vi "Configure Frequency Response Analysis Characteristics.vi"(5 "Enable Amplitude Ramp (F: Disable)":bool, 6 "Trace (4: Gain and Phase)":i32(ring)=4 items=["None", "All", "Gain", "Phase", "Gain and Phase"], 7 "Point Number (10: 10)":i32(ring)=10 items=["10"=10, "20"=20, "30"=30, "40"=40, "50"=50, "60"=60, "70"=70, "80"=80, "90"=90, "100"=100], 8 "error in (no error)":errorcluster, 9 "Single Frequency Value (1: 100 Hz)":i32(ring)=1 items=["20", "100", "1000", "10000", "100000", "1000000", "10000000", "2000000", "10"], 10 "Frequency Mode (0: Sweep)":i32(ring) items=["Sweep", "Single"], 11 "VISA resource name":refnum<visa-resource-name>) -> (0 "error out":errorcluster, 3 "VISA resource name out":refnum<visa-resource-name>)   [LabVIEW 2015, in "Agilent 2000 3000 X-Series.lvlib"]
doc: "Configure frequency response analysis feature.\n\n<b>Note:</b>\nThis VI is only applicable for 3000T, 4000, 6000 X-Series, 1000 X-Series after 1.10 firmware"
uses:
  Agilent 2000 3000 X-Series.lvlib
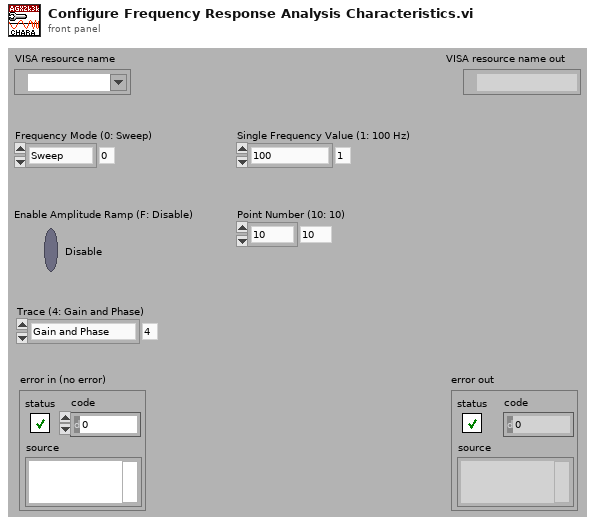
[diagram p1: front panel]
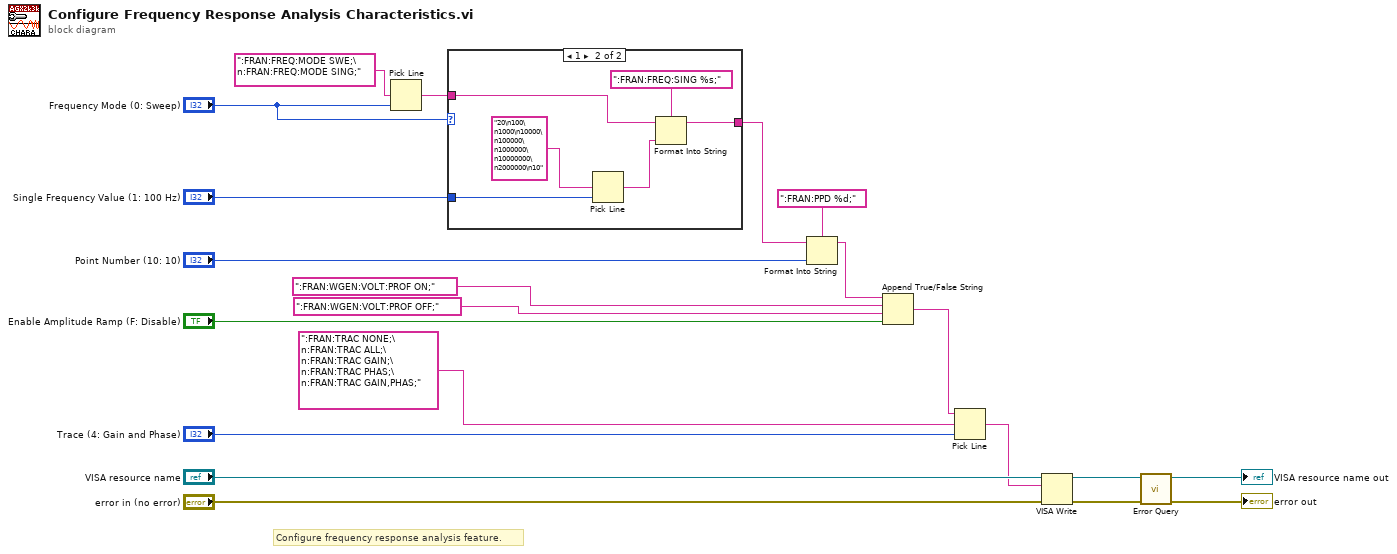
[diagram p0: block diagram]
diagram:
  # "Configure frequency response analysis feature."
  n1 = Pick Line(multi-line string=":FRAN:FREQ:MODE SWE;\n:FRAN:FREQ:MODE SING;", line index="Frequency Mode (0: Sweep)") -> (output string=w9:string)  [unwired: 1 in]
  n2 = case shown="1" "Frequency Mode (0: Sweep)" {
    tunnel: w9 -> [w22 w27]
    tunnel: [w22 w26] -> w8
    tunnel: "Single Frequency Value (1: 100 Hz)" -> [_ w23]
    frame 0, Default {
    }
    frame 1 {
      n3 = Pick Line(multi-line string="20\n100\n1000\n10000\n100000\n1000000\n10000000\n2000000\n10", line index=w23) -> (output string=w25:string)  [unwired: 1 in]
      n4 = Format Into String(format string=":FRAN:FREQ:SING %s;", initial string=w27, w25) -> (resulting string=w26:string)  [unwired: 1 in, 1 out]
    }
  }
  n5 = Format Into String(format string=":FRAN:PPD %d;", initial string=w8, "Point Number (10: 10)") -> (resulting string=w7:string)  [unwired: 1 in, 1 out]
  n6 = Append True/False String(1:"Enable Amplitude Ramp (F: Disable)", 2:":FRAN:WGEN:VOLT:PROF OFF;", 3:":FRAN:WGEN:VOLT:PROF ON;", 4:w7) -> (0:w4:string)
  n7 = Pick Line(string ("")=w4, multi-line string=":FRAN:TRAC NONE;\n:FRAN:TRAC ALL;\n:FRAN:TRAC GAIN;\n:FRAN:TRAC PHAS;\n:FRAN:TRAC GAIN,PHAS;", line index="Trace (4: Gain and Phase)") -> (output string=w3:string)
  n8 = VISA Write(VISA resource name="VISA resource name", write buffer=w3, error in (no error)="error in (no error)") -> (VISA resource name out=w14:refnum<visa-resource-name>, error out=w13:errorcluster)  [unwired: 1 out]
  n9 = call "Error Query.vi"("error in (no error)"=w13, "VISA resource name"=w14) -> ("error out"=→"error out":errorcluster, "VISA resource name out"=→"VISA resource name out":refnum<visa-resource-name>)  [unwired: 6 in, 2 out]
